vi "ComposeTitleBarString.vi"(1 "ProjectName":string, 2 "Application":string) -> (0 "TitleBar":string)   [LabVIEW 2014]
panel:
  out "FileName":string
  out "Application:Version Number":string
  out "FileVersion":string
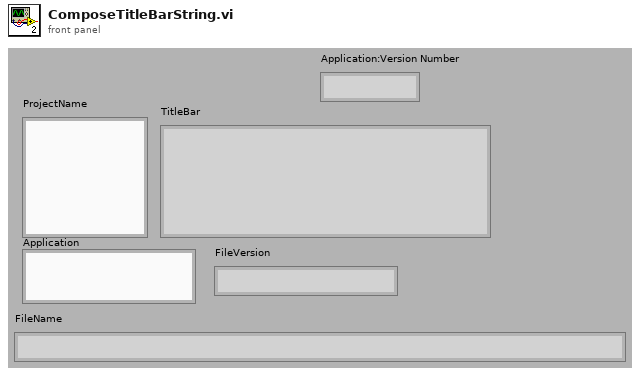
[diagram p1: front panel]
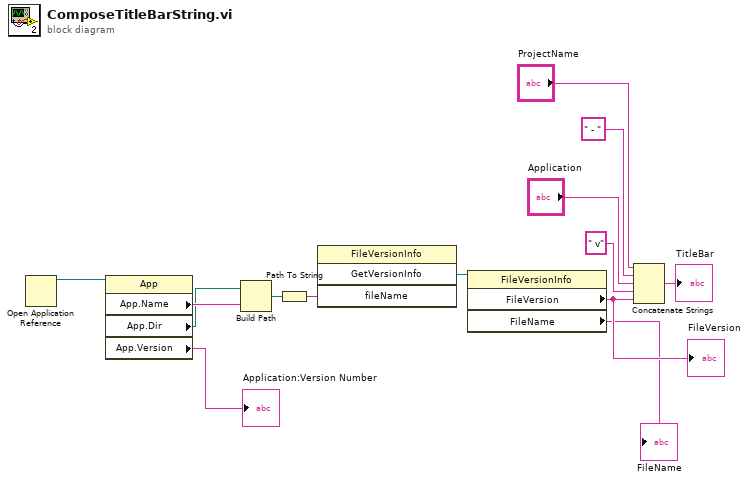
[diagram p0: block diagram]
diagram:
  n1 = Open Application Reference() -> (3:w7:refnum<vi>)  [unwired: 4 in, 1 out]
  n2 = property class="App"(reference=w7) -> ("App.Name"=w11:string, "App.Dir"=w10:path, "App.Version"=→"Application:Version Number":string)  [unwired: 1 in, 2 out]
  n3 = Build Path(base path=w10, name or relative path=w11) -> (appended path=w9:path)
  n4 = Path To String(path=w9) -> (string=w12:string)
  n5 = invoke class="FileVersionInfo" method="GetVersionInfo"("fileName"=w12) -> ("GetVersionInfo"=w6:refnum<k24>)  [unwired: 3 in, 3 out]
  n6 = property class="FileVersionInfo"(reference=w6) -> ("FileVersion"=w13:string, "FileName"=→"FileName":string)  [unwired: 1 in, 2 out]
  "FileVersion" <- w13
  n7 = Concatenate Strings("ProjectName", " - " ("string"), "Application", " v" ("string"), w13) -> (→"TitleBar":string)
